vi "Timer Page.vi"(11 "Main Panel":refnum<vi>) -> ()   [LabVIEW 2024, in "View.lvlib"]
uses:
  View.lvlib
  Support/Type Defs/Sequence Step--cluster.ctl
  Support/Type Defs/QMH Message--cluster.ctl
  Support/Type Defs/Timer Page Consumer Data--cluster.ctl
  Timer Page/Type Defs/Timer Helper Loop Data--cluster.ctl
panel:
  out "Elapsed Time":i16
  out "Timer Display":picture
  out "Sequence":T1[](array[typedef])
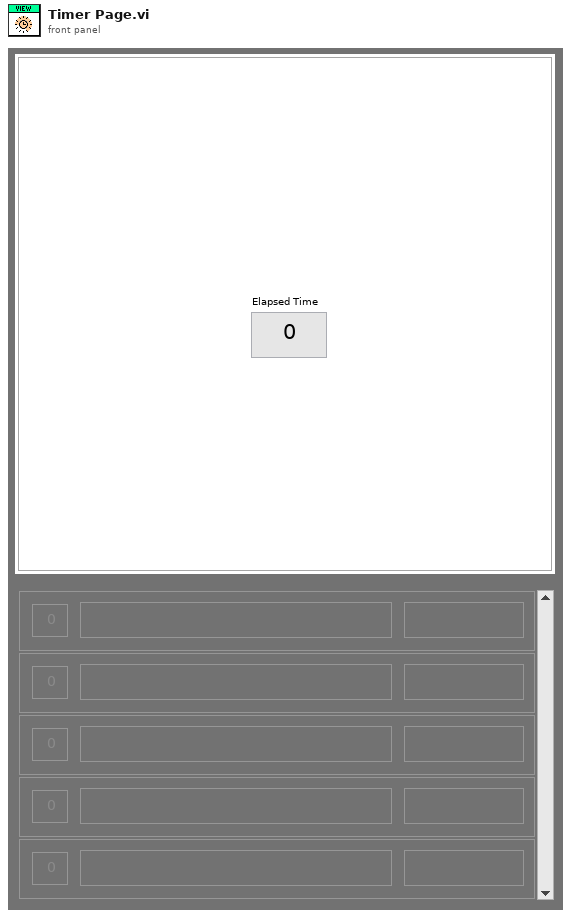
[diagram p1: front panel]
types:
  T1 = typedef "View.lvlib/Sequence Step--cluster.ctl" = cluster{"Step Number":dbl, "Step Name":string, "Duration":string}
  T2 = typedef "View.lvlib/Timer Helper Loop Data--cluster.ctl" = cluster{"Elapsed Time":dbl}
  T3 = typedef "View.lvlib/Timer Page Consumer Data--cluster.ctl" = cluster{"Panel Ref":refnum<vi>}
  T4 = typedef "View.lvlib/QMH Message--cluster.ctl" = cluster{"Message":string, "Message Data":variant}
  T5 = cluster{"Start Event":refnum<user-event>, "Pause Event":refnum<user-event>, "Stop Event":refnum<user-event>}
  T6 = cluster{"Width":u16, "Style":enum32{"Solid", "Dash", "Dot", "DashDot", "DashDotDot"}}
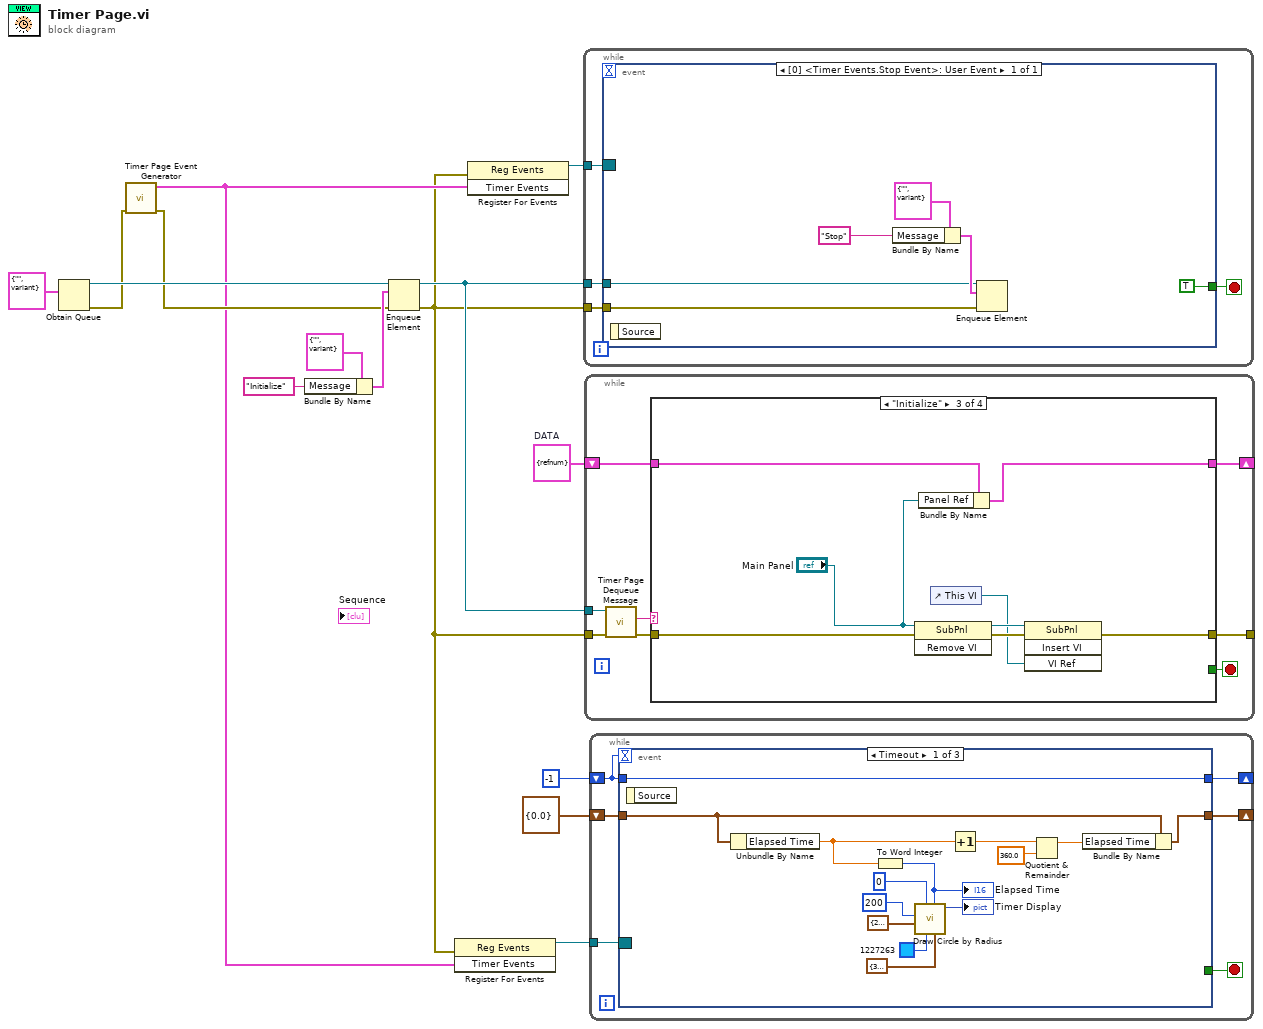
[diagram p0: block diagram]
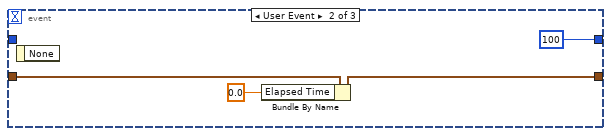
[diagram p2: hidden frame]
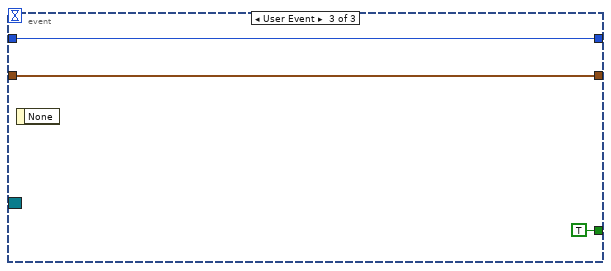
[diagram p3: hidden frame]
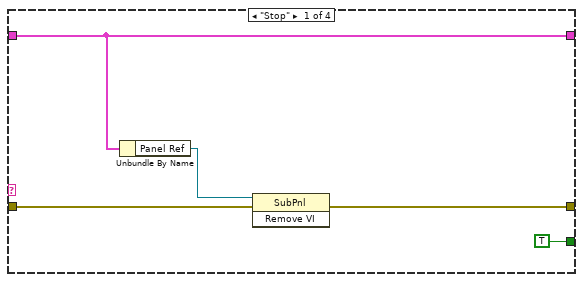
[diagram p4: hidden frame]
diagram:
  w9 = T3 {"Panel Ref"=refnum}  # DATA
  n1 = Obtain Queue(element data type=T4 {"Message"="", "Message Data"=variant} ("Message")) -> (queue out=w14:refnum<queue>, error out=w8:errorcluster)  [unwired: 4 in, 1 out]
  n2 = call "Timer Page Event Generator.vi"("error in"=w8) -> ("error out"=w7:errorcluster, "Timer Events"=w4:T5)  [unwired: 9 in]
  n3 = Bundle By Name(cluster=T4 {"Message"="", "Message Data"=variant} ("element"), "Message"="Initialize") -> (w11:T4)
  n4 = Enqueue Element(queue=w14, element=w11, error in (no error)=w7) -> (queue out=w13:refnum<queue>, error out=w1:errorcluster)  [unwired: 1 in, 1 out]
  n5 = register-events(error in=w1, w4) -> (reference out=w5:refnum<event-registration>)  [unwired: 1 in, 1 out]
  n6 = register-events(error in=w1, w4) -> (reference out=w6:refnum<event-registration>)  [unwired: 1 in, 1 out]
  n7 = while {
    tunnel: w13 -> [w19]
    tunnel: w1 -> [w18]
    tunnel: w6 -> [w16]
    stop <- w17 stop-if-true
    n8 = event shown="[0] <Timer Events.Stop Event>: User Event" {
      selector: w16 -> [_]
      dyn-events: _ -> [_]
      timeout: _ -> [_]
      tunnel: w19 -> [w23]
      tunnel: w18 -> [w22]
      tunnel: [TRUE] -> w17
      event User Event {
        n9 = event-data() -> ()  [unwired: 1 in, 1 out]
        n10 = Bundle By Name(cluster=T4 {"Message"="", "Message Data"=variant} ("element"), "Message"="Stop") -> (w24:T4)
        n11 = Enqueue Element(queue=w23, element=w24, error in (no error)=w22) -> ()  [unwired: 1 in, 3 out]
      }
    }
  }
  n12 = while {
    tunnel: w13 -> [w27]
    tunnel: w1 -> [w29]
    shift-right: [w32] -> _
    shift-left: w9 -> [w33]
    tunnel: [w31] -> _
    stop <- w30 stop-if-true
    n13 = call "Timer Page Dequeue Message.vi"("error in (no error)"=w29, "Queue in"=w27) -> ("error out"=w28:errorcluster, "Message"=w26:string)  [unwired: 7 in, 1 out]
    n14 = case shown="\"Initialize\"" w26 {
      tunnel: w33 -> [w35 w40 w45 w50]
      tunnel: [w35 w40 w44 w50] -> w32
      tunnel: w28 -> [w38 w39 w43 w49]
      tunnel: [w36 w39 w42 w49] -> w31
      tunnel: [TRUE _ _ _] -> w30
      frame "Stop" {
        n15 = Unbundle By Name(w35) -> ("Panel Ref"=w34:refnum<vi>)
        n16 = invoke class="SubPnl" method="Remove VI"(reference=w34, error in=w38) -> (error out=w36:errorcluster)  [unwired: 1 in, 2 out]
      }
      frame Default {
      }
      frame "Initialize" {
        n17 = invoke class="SubPnl" method="Remove VI"(reference="Main Panel", error in=w43) -> (reference out=w47:refnum<vi>, error out=w48:errorcluster)  [unwired: 1 in, 1 out]
        n18 = Bundle By Name(cluster=w45, "Panel Ref"="Main Panel") -> (w44:T3)
        n19 = control-ref of="This VI"() -> (w46:refnum<vi>)
        n20 = invoke class="SubPnl" method="Insert VI"(reference=w47, error in=w48, "VI Ref"=w46) -> (error out=w42:errorcluster)  [unwired: 1 in, 3 out]
      }
      frame "Start Module" {
      }
    }
  }
  n21 = while {
    tunnel: w5 -> [w56]
    shift-right: [w54] -> _
    shift-left: -1 -> [w55]
    shift-right: [w52] -> _
    shift-left: T2 {"Elapsed Time"=0.0} ("DATA") -> [w53]
    stop <- w51 stop-if-true
    n22 = event shown="[0] Timeout" {
      selector: w56 -> [_ _ _]
      dyn-events: _ -> [_ _ _]
      timeout: w55 -> [_ _ _]
      tunnel: w55 -> [w70 _ w75]
      tunnel: [w70 100 w75] -> w54
      tunnel: w53 -> [w64 w73 w76]
      tunnel: [w63 w72 w76] -> w52
      tunnel: [_ _ TRUE] -> w51
      event Timeout {
        n23 = event-data() -> ()  [unwired: 1 in, 1 out]
        n24 = Unbundle By Name(w64) -> ("Elapsed Time"=w62:dbl)
        n25 = To Word Integer(number=w62) -> (16bit integer=w57:i16)
        "Elapsed Time" <- w57
        n26 = call <vilib>:"Draw Circle by Radius.vi"("pen"=T6 {"Width"=35, "Style"=enum."Solid"}, "arc size(360)"=w57, "color(black)"=u32 1227263, "start angle(0)"=i16 0, "pixel center"=cluster{"horizontal":i16, "vertical":i16} {"horizontal"=260, "vertical"=270}, "radius"=i16 200) -> ("new picture"=→"Timer Display":picture)  [unwired: 5 in]
        n27 = Increment(x=w62) -> (x+1=w61:dbl)
        n28 = Quotient & Remainder(x=w61, y=360.0) -> (x-y*floor(x/y)=w60:dbl)  [unwired: 1 out]
        n29 = Bundle By Name(cluster=w64, "Elapsed Time"=w60) -> (w63:T2)
      }
      event User Event {
        n30 = event-data() -> ()  [unwired: 1 in, 1 out]
        n31 = Bundle By Name(cluster=w73, "Elapsed Time"=0.0) -> (w72:T2)
      }
      event User Event {
        n32 = event-data() -> ()  [unwired: 1 in, 1 out]
      }
    }
  }
